vi "CalibrationDataCollection.vi"() -> ()   [LabVIEW 2020]
doc: "Use this template to build a producer/consumer design pattern. Use this template when you need to execute a process, such as data analysis, when a data source, such as a triggered acquisition, produces data at an uneven rate and you need to execute the process when the data becomes available.\n------------------------------------\nAuther: Koji Ohashi\nCopyright (c) 2020 Japan LabVIEW Users Group, Volunteer members.\nThis VI is released under the MIT License.\nhttp://opensource.org/licenses/mit-license.php\n------------------------------------"
uses:
  FSRCalibrationDataCollection Folder/For fsr type def.ctl
  <vilib>/Platform/TimedLoop/XDataNode/timing_clust.ctl
  <vilib>/Platform/TimedLoop/XDataNode/nitl_modes.ctl
  <vilib>/Platform/TimedLoop/XDataNode/wakeup.ctl
  <vilib>/Instr/_visa.llb/VISA Configure Serial Port (Instr).vi
  <vilib>/platform/TimedLoop/XDataNode/XDataNode.xnode
  <vilib>/Platform/TimedLoop/XDataNode/XDNodeRunTimeDep.lvlib
panel:
  out "Collecting":bool
  in  "Timer [ms]":u32
  out "On Time [ms]":u32
  out "millisecond timer":u32
  in  "Weight":T1(ring)
  out "Vout F1":dbl(slide) scale=-100.0..100.0
  in  "?":bool
  in  "Weight":string
  in  "Path":path=path "C:/Users/rsKite/Documents/FSR DATA"
  in  "Trial":string caption="Participant Name (FirstLast)"
  out "File Name":string
  out "Vout F3":dbl(slide) scale=0.0..2000.0
  out "Vout F2":dbl(slide) scale=0.0..2000.0
  out "Status":string
  in  "?":bool
  in  "VISA resource name":refnum<visa-resource-name>="COM1"
  in  "stop":bool
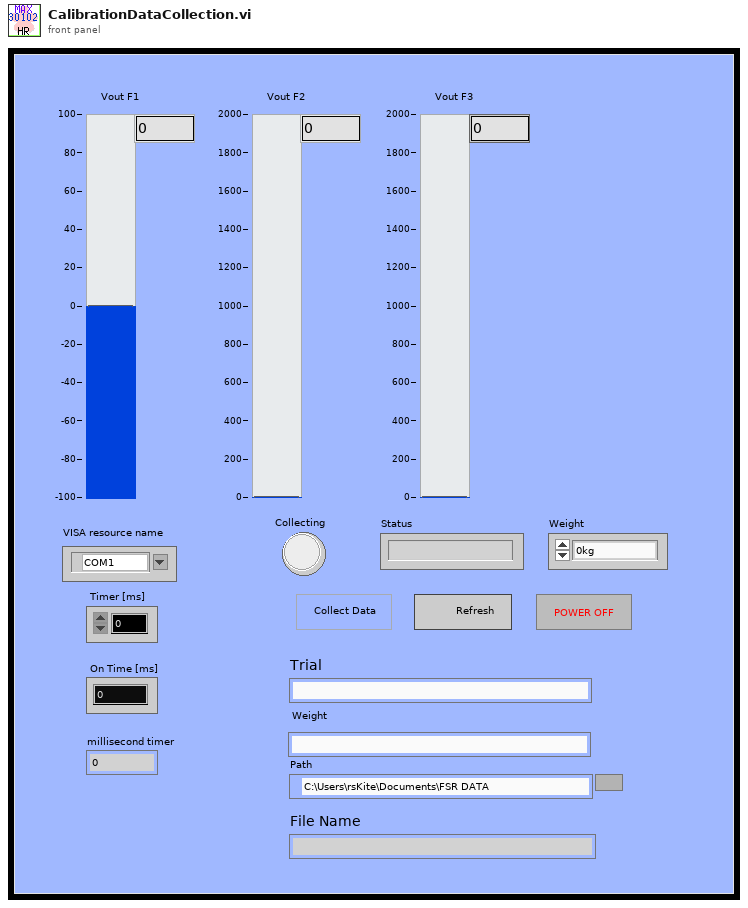
[diagram p1: front panel]
types:
  T1 = enum16{"0kg", "0.1kg", "0.2kg", "0.3kg", "0.4kg", "0.5kg", "0.6kg", "0.7kg", "0.8kg", "0.9kg", "1kg", "1.1kg", "1.2kg", "1.3kg", "1.4kg", "1.5kg", "1.6kg", "1.7kg", "1.8kg", "1.9kg", "2.0kg"}
  T2 = enum16{"open", "replace", "create", "open or create", "replace or create", "replace or create with confirmation"}
  T3 = typedef "For fsr type def.ctl" = enum16{"Create/Replace File", "Waiting Room", "Collect Data", "Write Data", "Close File", "Reinit"}
  T4 = typedef "XDNodeRunTimeDep.lvlib/timing_clust.ctl" = cluster{"Expected End [f-1]":u64, "Actual End [f-1]":u64, "Finished Late? [f-1]":bool, "Expected End [i-1]":u64, "Actual End [i-1]":u64, "Finished Late? [i-1]":bool, "Expected Start [i]":u64, "Actual Start [i]":u64, "Expected Start [f]":u64, "Actual Start [f]":u64, "Source Name":string, "Structure Name":string, "Period":i64, "Deadline":i64, "Offset":i64, "Start":i64, "Priority":i32, "Timeout":i32, "Mode":T5, "Wakeup Reason":T6, "Error":errorcluster, "Source Type":string, "Secondary Source Type":string, "Global End Time":u64, "Global Start Time":u64, "Frame Duration":u64, "Iteration Duration":u64, "Assigned CPU":i32, "I/O Scan Engine Mode":u32}
  T5 = typedef "XDNodeRunTimeDep.lvlib/nitl_modes.ctl" = enum32{"No Change", "Process missed periods, maintain original phase", "Discard missed periods, maintain original phase", "Process missed periods, ignore original phase", "Discard missed periods, ignore original phase"}
  T6 = typedef "XDNodeRunTimeDep.lvlib/wakeup.ctl" = enum32{"Normal", "Aborted", "Asynchronous wakeup", "Timing source error", "Timed loop error", "Timeout"}
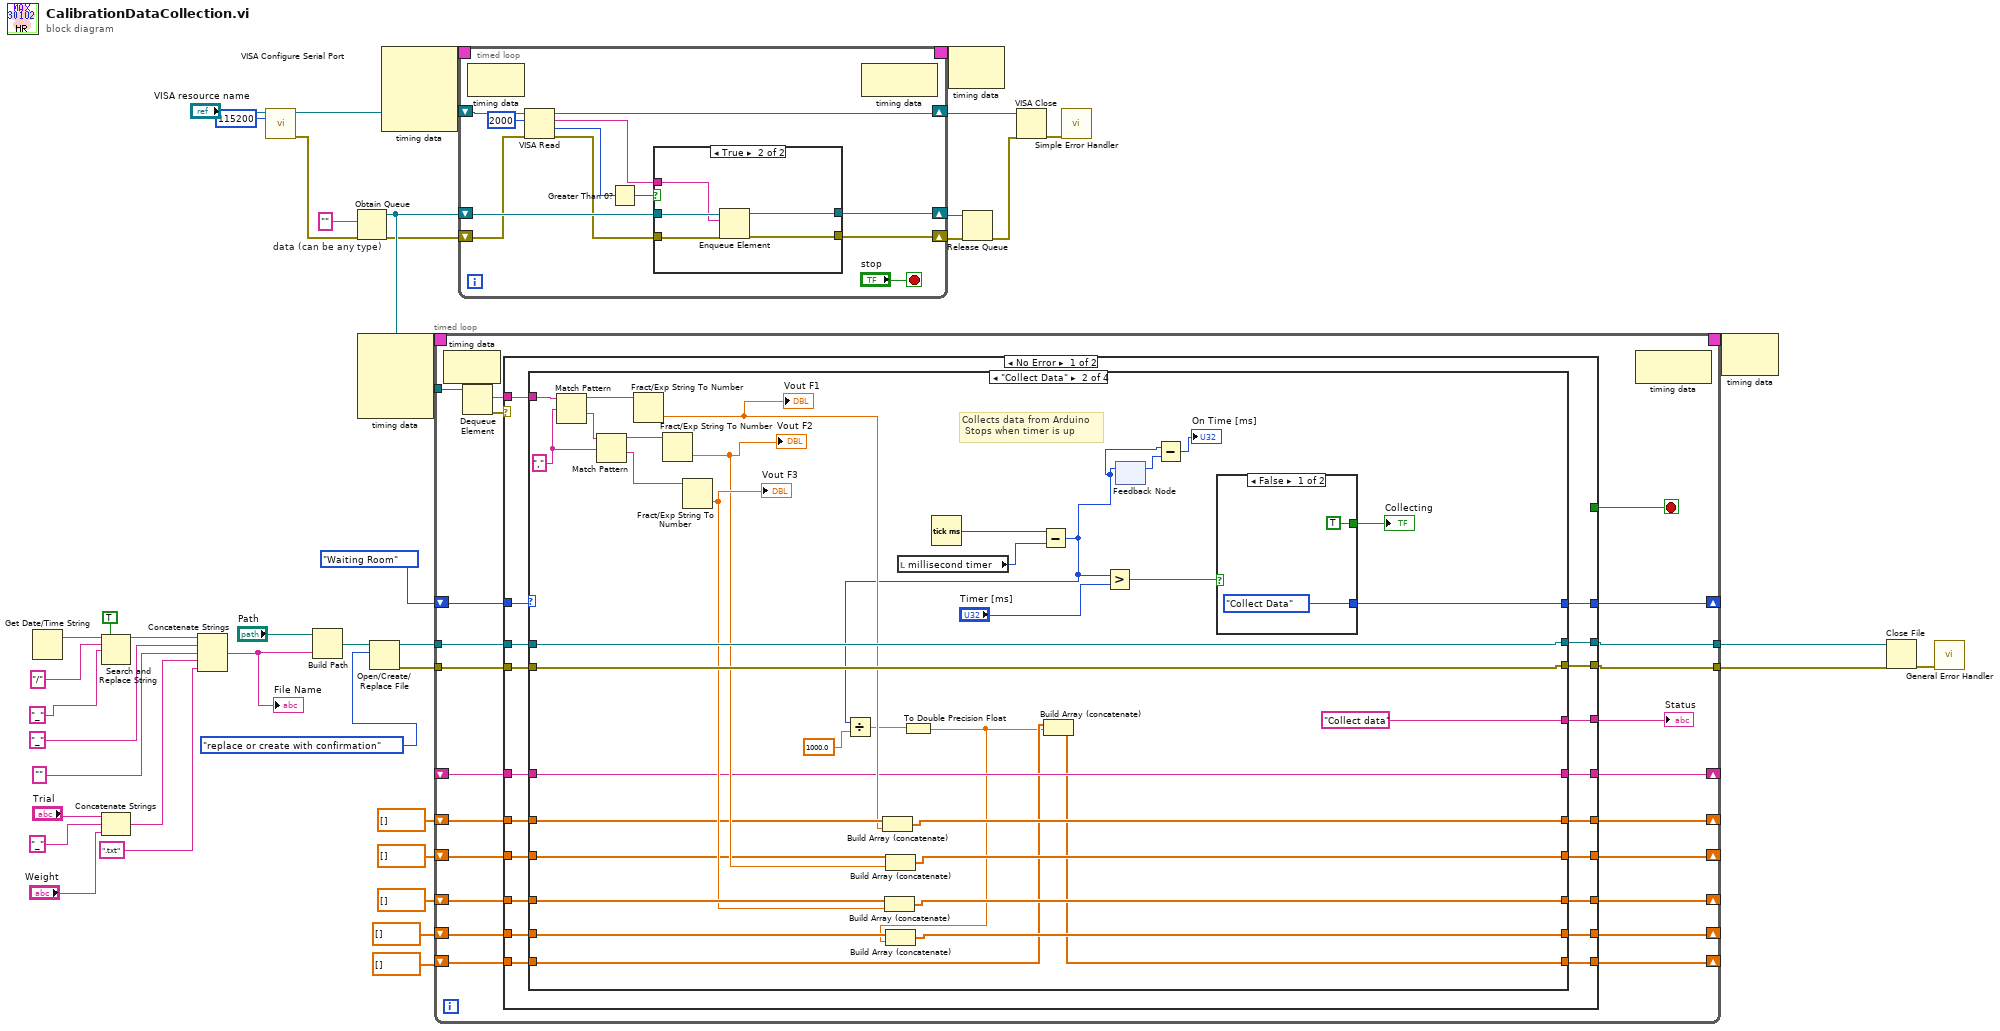
[diagram p0: block diagram]
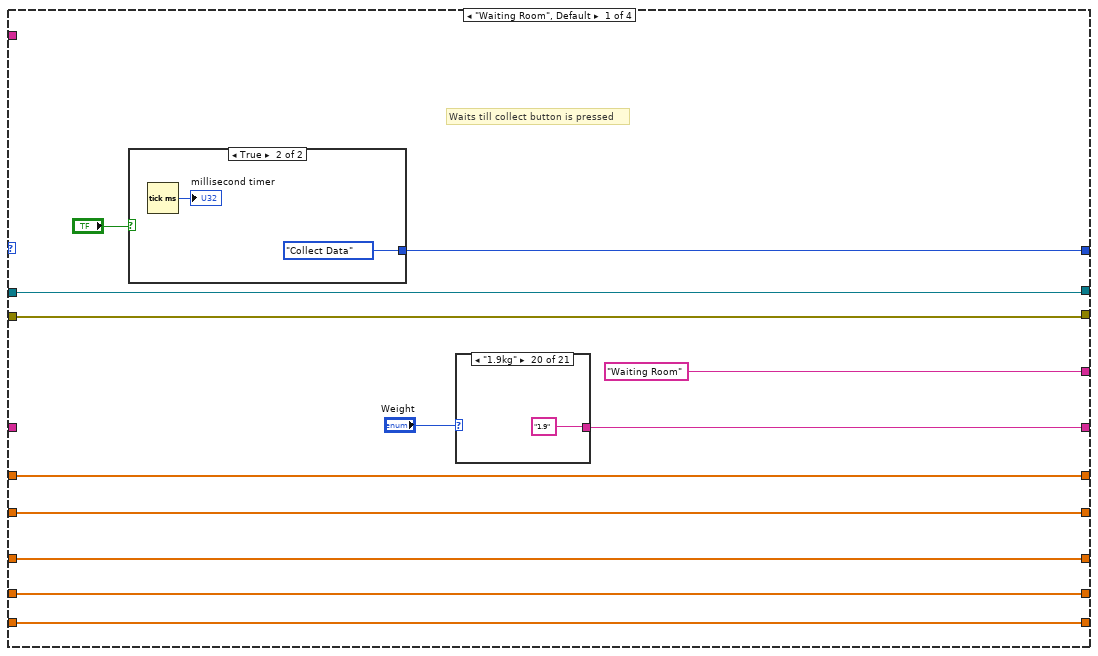
[diagram p2: hidden frame]
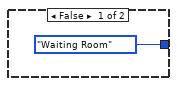
[diagram p3: hidden frame]
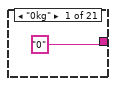
[diagram p4: hidden frame]
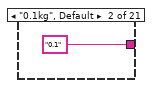
[diagram p5: hidden frame]
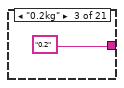
[diagram p6: hidden frame]
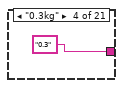
[diagram p7: hidden frame]
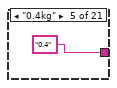
[diagram p8: hidden frame]
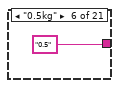
[diagram p9: hidden frame]
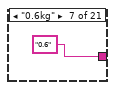
[diagram p10: hidden frame]
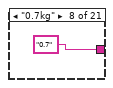
[diagram p11: hidden frame]
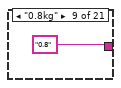
[diagram p12: hidden frame]
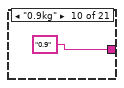
[diagram p13: hidden frame]
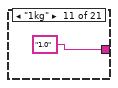
[diagram p14: hidden frame]
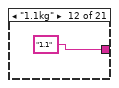
[diagram p15: hidden frame]
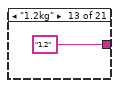
[diagram p16: hidden frame]
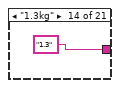
[diagram p17: hidden frame]
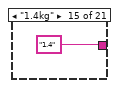
[diagram p18: hidden frame]
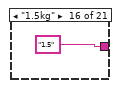
[diagram p19: hidden frame]
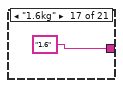
[diagram p20: hidden frame]
diagram:
  w39 = ""  # data (can be any type)
  n1 = Get Date/Time String() -> (date string=w30:string)  [unwired: 3 in, 1 out]
  n2 = Search and Replace String(replace all?=TRUE ("replace all? (F)"), input string=w30, search string="/", replace string="_" ("replace string (\"\")")) -> (result string=w28:string)  [unwired: 4 in, 3 out]
  n3 = Concatenate Strings("Trial", "_" ("string"), "Weight") -> (w29:string)
  n4 = Concatenate Strings(w28, "_" ("string"), "" ("string"), w29, ".txt" ("string")) -> (w26:string)
  "File Name" <- w26
  n5 = call-poly "VISA Configure Serial Port"("VISA resource name"="VISA resource name", "baud rate (9600)"=u32 115200) -> ("VISA resource name out"=w37:refnum<visa-resource-name>, "error out"=w34:errorcluster)  [unwired: 8 in, 4 out]
  n6 = Build Path(base path="Path", name or relative path=w26) -> (appended path=w15:path)
  n7 = Obtain Queue(element data type=w39, error in (no error)=w34) -> (queue out=w43:refnum<queue>, error out=w42:errorcluster)  [unwired: 3 in, 1 out]
  n8 = node-c288() -> (w2:T4)  [unwired: 4 in]
  n9 = Open/Create/Replace File(file path (use dialog)=w15, operation (0:open)=T2."replace or create with confirmation") -> (refnum out=w13:refnum<file>, error out=w12:errorcluster)  [unwired: 4 in, 1 out]
  n10 = node-c288() -> (w4:T4)  [unwired: 4 in]
  n11 = timed-loop {
    tunnel: w43 -> [w66]
    shift-right: [w60] -> _
    shift-left: For_fsr_type_def."Waiting Room" -> [w61]
    tunnel: w13 -> [w59]
    tunnel: w12 -> [w58]
    tunnel: [w57] -> w11
    tunnel: [w56] -> w10
    shift-right: [w52] -> _
    shift-left: dbl[] [] -> [w53]
    shift-right: [w54] -> _
    shift-left: dbl[] [] -> [w55]
    shift-right: [w50] -> _
    shift-left: dbl[] [] -> [w51]
    shift-right: [w48] -> _
    shift-left: _ -> [w49]
    shift-right: [w46] -> _
    shift-left: dbl[] [] -> [w47]
    shift-right: [w45] -> _
    shift-left: dbl[] [] -> [w44]
    timing: w2 -> [_]
    timing-out: [_] -> w1
    stop <- w63 stop-if-true
    n12 = node-c288() -> ()  [unwired: 1 in, 1 out]
    n13 = Dequeue Element(queue=w66) -> (element=w64:string, error out=w65:errorcluster)  [unwired: 2 in, 2 out]
    n14 = case shown="No Error" w65 {
      tunnel: w64 -> [w86 _]
      tunnel: [_ TRUE] -> w63
      tunnel: [w85 "Error or POWER OFF"] -> w62
      tunnel: w61 -> [w88 _]
      tunnel: [w87 For_fsr_type_def."Waiting Room"] -> w60
      tunnel: w59 -> [w84 w230]
      tunnel: w58 -> [w83 w229]
      tunnel: [w82 w230] -> w57
      tunnel: [w81 w229] -> w56
      tunnel: w55 -> [w80 w226]
      tunnel: [w79 w226] -> w54
      tunnel: w53 -> [w78 w227]
      tunnel: [w77 w227] -> w52
      tunnel: w51 -> [w76 w228]
      tunnel: [w75 w228] -> w50
      tunnel: w49 -> [w74 w225]
      tunnel: [w73 w225] -> w48
      tunnel: w47 -> [w72 w224]
      tunnel: [w71 w224] -> w46
      tunnel: [w70 w223] -> w45
      tunnel: w44 -> [w69 w223]
      frame No Error {
        n15 = case shown="\"Collect Data\"" w88 {
          tunnel: [w92 w139 For_fsr_type_def."Reinit" w205] -> w87
          tunnel: w86 -> [_ w158 _ _]
          tunnel: ["Waiting Room" "Collect data" "Write Data" "Reinit"] -> w85
          tunnel: w84 -> [w99 w156 w183 w207]
          tunnel: w83 -> [w98 w155 w182 w206]
          tunnel: [w99 w156 w181 w207] -> w82
          tunnel: [w98 w155 w180 w206] -> w81
          tunnel: w80 -> [w95 w152 w172 w199]
          tunnel: [w95 w136 w172 w202] -> w79
          tunnel: w78 -> [w96 w149 w173 w200]
          tunnel: [w96 w147 w173 w203] -> w77
          tunnel: w76 -> [w97 w148 w174 w201]
          tunnel: [w97 w146 w174 w204] -> w75
          tunnel: [w94 w144 w177 w196] -> w73
          tunnel: w74 -> [_ w144 w177 w197]
          tunnel: w72 -> [w90 w135 w171 w195]
          tunnel: [w90 w134 w171 w194] -> w71
          tunnel: [w89 w131 w170 w192] -> w70
          tunnel: w69 -> [w89 w130 w170 w193]
          frame "Waiting Room", Default {
            # "Waits till collect button is pressed"
            n16 = case shown="True" "?" {
              tunnel: [For_fsr_type_def."Waiting Room" For_fsr_type_def."Collect Data"] -> w92
              frame False {
              }
              frame True {
                n17 = Tick Count (ms)() -> (millisecond timer value=→"millisecond timer":u32)
              }
            }
            n18 = case shown="\"1.9kg\"" "Weight" {
              tunnel: ["0" "0.1" "0.2" "0.3" "0.4" "0.5" "0.6" "0.7" "0.8" "0.9" "1.0" "1.1" "1.2" "1.3" "1.4" "1.5" "1.6" "1.7" "1.8" "1.9" "2.0"] -> w94
              frame "0kg" {
              }
              frame "0.1kg", Default {
              }
              frame "0.2kg" {
              }
              frame "0.3kg" {
              }
              frame "0.4kg" {
              }
              frame "0.5kg" {
              }
              frame "0.6kg" {
              }
              frame "0.7kg" {
              }
              frame "0.8kg" {
              }
              frame "0.9kg" {
              }
              frame "1kg" {
              }
              frame "1.1kg" {
              }
              frame "1.2kg" {
              }
              frame "1.3kg" {
              }
              frame "1.4kg" {
              }
              frame "1.5kg" {
              }
              frame "1.6kg" {
              }
              frame "1.7kg" {
              }
              frame "1.8kg" {
              }
              frame "1.9kg" {
              }
              frame "2.0kg" {
              }
            }
          }
          frame "Collect Data" {
            w137 = ","
            # "Collects data from Arduino\n Stops when timer is up"
            n19 = Match Pattern(string=w158, regular expression=w137) -> (before substring=w154:string, after substring=w153:string)  [unwired: 1 in, 2 out]
            n20 = Match Pattern(string=w153, regular expression=w137) -> (before substring=w157:string, after substring=w126:string)  [unwired: 1 in, 2 out]
            n21 = Fract/Exp String To Number(string=w154) -> (number=w145:dbl)  [unwired: 3 in, 1 out]
            "Vout F1" <- w145
            n22 = Fract/Exp String To Number(string=w157) -> (number=w150:dbl)  [unwired: 3 in, 1 out]
            "Vout F2" <- w150
            n23 = Fract/Exp String To Number(string=w126) -> (number=w151:dbl)  [unwired: 3 in, 1 out]
            "Vout F3" <- w151
            n24 = Build Array (concatenate)(w148, w145) -> (w146:dbl[])
            n25 = Build Array (concatenate)(w152, w151) -> (w136:dbl[])
            n26 = Build Array (concatenate)(w149, w150) -> (w147:dbl[])
            n27 = local read "millisecond timer"() -> (w141:u32)
            n28 = Tick Count (ms)() -> (millisecond timer value=w143:u32)
            n29 = Subtract(x=w143, y=w141) -> (x-y=w128:u32)
            n30 = Divide(x=w128, y=1000.0) -> (x/y=w132:dbl)
            n31 = To Double Precision Float(number=w132) -> (double precision float=w125:dbl)
            n32 = Build Array (concatenate)(w135, w125) -> (w134:dbl[])
            n33 = Build Array (concatenate)(w130, w125) -> (w131:dbl[])
            n34 = Greater?(x=w128, y="Timer [ms]") -> (0:w138:bool)
            n35 = feedback-in #1(w128) -> ()
            n36 = feedback #1() -> (w129:u32)  [unwired: 1 in]
            n37 = Subtract(x=w128, y=w129) -> (x-y=→"On Time [ms]":u32)
            n38 = case shown="False" w138 {
              tunnel: [TRUE FALSE] -> w140
              tunnel: [For_fsr_type_def."Collect Data" For_fsr_type_def."Write Data"] -> w139
              frame False {
              }
              frame True {
              }
            }
            "Collecting" <- w140
          }
          frame "Write Data" {
            # "Puts the data to a spreadsheet and writes it to the file"
            n39 = Build Array(w174, w173, w172, w171, w170) -> (w168:dbl[][])
            n40 = Transpose Matrix(1:w168) -> (0:w169:dbl[][])
            n41 = Array To Spreadsheet String(array=w169, 3:"%5.3f" ("format string")) -> (spreadsheet string=w166:string)  [unwired: 1 in]
            n42 = Concatenate Strings(w177, "\r\n", "F1", "\t", "F2", "\t", "F3", "\t", "F4", "\t", "time", "\r\n", w166) -> (w188:string)
            n43 = Write to Text File(file (use dialog)=w183, text=w188, error in=w182) -> (refnum out=w181:refnum<file>, error out=w180:errorcluster)  [unwired: 1 in, 1 out]
          }
          frame "Reinit" {
            # "Clears data previously collected"
            n44 = case shown="True" "?" {
              tunnel: [For_fsr_type_def."Reinit" For_fsr_type_def."Waiting Room"] -> w205
              tunnel: [w215 dbl[] []] -> w204
              tunnel: [w214 dbl[] []] -> w203
              tunnel: [w213 dbl[] []] -> w202
              tunnel: w201 -> [w215 _]
              tunnel: w200 -> [w214 _]
              tunnel: w199 -> [w213 _]
              tunnel: w197 -> [w211 _]
              tunnel: [w211 ""] -> w196
              tunnel: w195 -> [w210 _]
              tunnel: [w210 dbl[] []] -> w194
              tunnel: w193 -> [w209 _]
              tunnel: [w209 dbl[] []] -> w192
              frame False {
              }
              frame True {
              }
            }
          }
        }
      }
      frame Error {
      }
    }
    "Status" <- w62
    n45 = node-c288() -> ()  [unwired: 1 in, 1 out]
  }
  n46 = timed-loop {
    shift-right: [w242] -> w40
    shift-left: w42 -> [w237]
    shift-right: [w243] -> w41
    shift-left: w43 -> [w244]
    shift-right: [w241] -> w35
    shift-left: w37 -> [w235]
    timing: w4 -> [_]
    timing-out: [_] -> w3
    stop <- "stop" stop-if-true
    n47 = node-c288() -> ()  [unwired: 1 in, 1 out]
    n48 = VISA Read(VISA resource name=w235, byte count=u32 2000, error in (no error)=w237) -> (VISA resource name out=w241:refnum<visa-resource-name>, read buffer=w238:string, return count=w240:u32, error out=w236:errorcluster)
    n49 = Greater Than 0?(x=w240) -> (x > 0?=w239:bool)
    n50 = case shown="True" w239 {
      tunnel: w244 -> [w249 w254]
      tunnel: [w249 w253] -> w243
      tunnel: w236 -> [w248 w252]
      tunnel: [w248 w251] -> w242
      tunnel: w238 -> [_ w250]
      frame False {
      }
      frame True {
        n51 = Enqueue Element(queue=w254, element=w250, error in (no error)=w252) -> (queue out=w253:refnum<queue>, error out=w251:errorcluster)  [unwired: 1 in, 1 out]
      }
    }
    n52 = node-c288() -> ()  [unwired: 1 in, 1 out]
  }
  n53 = node-c288(w3) -> ()  [unwired: 1 out]
  n54 = Release Queue(queue=w41, error in (no error)=w40) -> (error out=w33:errorcluster)  [unwired: 1 in, 2 out]
  n55 = VISA Close(VISA resource name=w35, error in (no error)=w33) -> (error out=w36:errorcluster)
  n56 = call <vilib>:"Simple Error Handler.vi"("error in (no error)"=w36) -> ()  [unwired: 1 in, 8 out]
  n57 = node-c288(w1) -> ()  [unwired: 1 out]
  n58 = Close File(refnum=w11, error in=w10) -> (error out=w14:errorcluster)  [unwired: 1 out]
  n59 = call <vilib>:"General Error Handler.vi"("error in (no error)"=w14) -> ()  [unwired: 10 in, 5 out]
